vi "Renew Controls Attribute.vi"(8 "error in (no error)":errorcluster, 10 "Control Refs":refnum<vi>[](array[refnum]), 11 "UIConfiguration in":refnum<class "UIConfiguration.lvclass">) -> (0 "error out":errorcluster, 3 "UIConfiguration out":refnum<class "UIConfiguration.lvclass">)   [LabVIEW 2015, in "UIConfiguration.lvclass"]
uses:
  UIConfiguration.lvclass
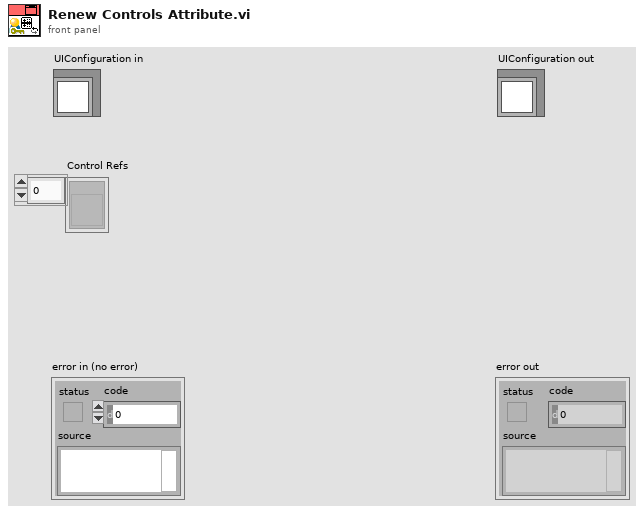
[diagram p1: front panel]
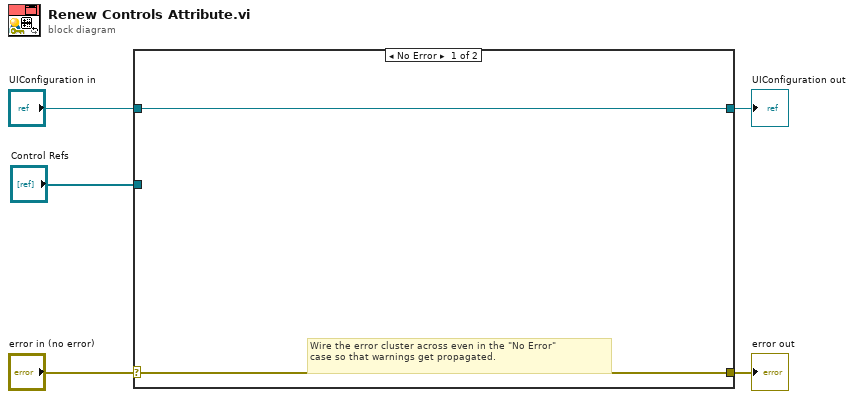
[diagram p0: block diagram]
diagram:
  n1 = case shown="No Error" "error in (no error)" {
    selector: "error in (no error)" -> [w6 w9]
    tunnel: [w6 w9] -> w4
    tunnel: [w7 w8] -> w2
    tunnel: "UIConfiguration in" -> [w7 w8]
    tunnel: "Control Refs" -> [_ _]
    frame No Error {
      # "Wire the error cluster across even in the \"No Error\"\ncase so that warnings get propagated."
    }
    frame Error {
    }
  }
  "error out" <- w4
  "UIConfiguration out" <- w2
